vi "BatchLoad DataBuffer.vi"(0 "Display#":u16(slide)=1 min=1 max=1 step=1 scale=1.0..1.1, 7 "File Info Buffer Init":T1[](array[typedef]) {"CCD Parameters"."dt or s" format="%#.6f"; "CCD Parameters"."Repetition" min=1; "CCD Parameters"."Offset" format="%#.2f"; "CCD Parameters"."Exposure Time (s)" min=0.02 max=6000.0 format="%#.2f"; "Center nm" format="%.2f"; "Temperature (K)" format="%.2f"; "Field (T)" format="%.2f"}, 11 "Y Array In":dbl[][](array[numeric])=array1025x10[10250 elements] format="%.2f") -> (3 "File Info Out":T1={"FilePath"=path "/DATA/Labview Items", "Field (T)"=55.0, "Temperature (K)"=77.0, "X-Axis"=enum."nm", "Center nm"=55.0, "Current Grating Density"=enum."600", "CCD Parameters"={"Exposure Time (s)"=0.2, "Offset"=0.0, "BkgrdCrct"=FALSE, "Shutter"=FALSE, "Mode"=enum."Regular", "Repetition"=4, "dt or s"=0.0}, "Operation Mode"=enum."NML Data Acquisition", "Exp Index"=0, "Index_repetition"=0, "Index"=0, "Current Detector"=enum."CCD-1024x256"} {"CCD Parameters"."dt or s" format="%#.6f"; "CCD Parameters"."Repetition" min=1; "CCD Parameters"."Offset" format="%#.2f"; "CCD Parameters"."Exposure Time (s)" min=0.02 max=6000.0 format="%#.2f"; "Center nm" format="%.2f"; "Temperature (K)" format="%.2f"; "Field (T)" format="%.2f"}, 4 "X-Data out":dbl[](array[numeric]) format="%.2f", 6 "Y-Data out":dbl[](array[numeric]) format="%.2f", 8 "X-Axis":i32(ring)=1 items=["Point #", "nm", "eV", "meV", "cm-1"], 10 "File Info Buffer Out":T1[](array[typedef]) {"CCD Parameters"."dt or s" format="%#.6f"; "CCD Parameters"."Repetition" min=1; "CCD Parameters"."Offset" format="%#.2f"; "CCD Parameters"."Exposure Time (s)" min=0.02 max=6000.0 format="%#.2f"; "Center nm" format="%.2f"; "Temperature (K)" format="%.2f"; "Field (T)" format="%.2f"}, 14 "Continue?":bool, 15 "Y Array Out":dbl[][](array[numeric]) format="%.2f")   [LabVIEW 2019]
doc: "Write (FIFO) or retrieve (LIFO) data from the buffer.\n\nWhen write to the buffer, set the desired \"Buffer Size\" and run the VI several iterations. Notice that initially, the buffer grows to reach \"Buffer Size\" and then the input data flows from the last buffer element through to the zero element on each iteration (First In, First Out).\n\nWhen read from the buffer, set the Read# to the nth previous input data, i.e. counting reversely, with the most recent input counted as the 1st readout. If the input is out of current buffer size, an error is returned. (Last In, First Out)"
uses:
  Globals and TypeDefs/Type Definitions.llb/FileInfoParameter.ctt
  Globals and TypeDefs/Type Definitions.llb/Wavelength Unit.ctt
  Globals and TypeDefs/Type Definitions.llb/McPherson Grating Density.ctl
  Globals and TypeDefs/Type Definitions.llb/CCDParameter.ctt
  Globals and TypeDefs/Type Definitions.llb/OperationMode.ctt
  Globals and TypeDefs/Type Definitions.llb/ListOfDetectors.ctt
  File and save/X-Axis_Generator_morph.vi
panel:
  in  "End #":i16
  in  "Start #":i16
  in  "continue2":bool=TRUE
  in  "Speed":u16(slide)=100 min=50 max=5000 step=50 scale=10.0..5000.0
  in  "Movie":bool
  out "File Contents":string
  in  "WL unit":i32(ring)=1 items=["Wavelength", "nm", "eV", "meV", "cm-1"]
  in  "Continue?":bool
  in  "Cancel":bool
  out "File Path":path
  out "?":T7(graph)
  # "Latest"
  # "Erliest"
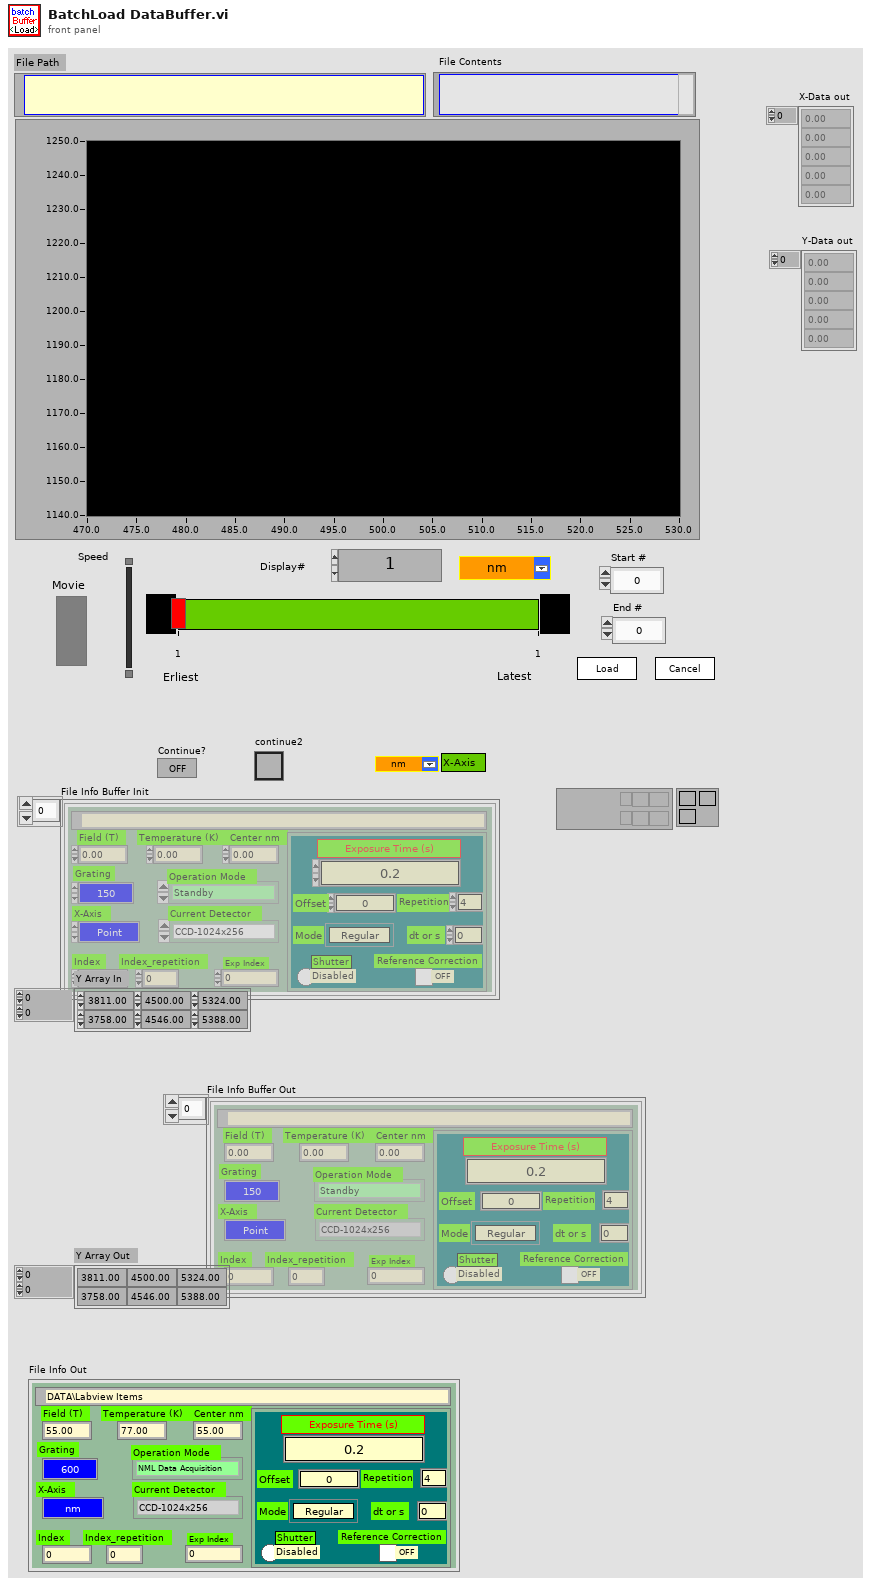
[diagram p1: front panel]
types:
  T1 = typedef "FileInfoParameter.ctt" = cluster{"FilePath":path, "Field (T)":dbl, "Temperature (K)":dbl, "X-Axis":T2, "Center nm":dbl, "Current Grating Density":T3, "CCD Parameters":T4, "Operation Mode":T5, "Exp Index":u32, "Index_repetition":u16, "Index":u16, "Current Detector":T6}
  T2 = typedef "Wavelength Unit.ctt" = enum8{"Point", "nm", "eV", "meV", "cm_1"}
  T3 = typedef "McPherson Grating Density.ctl" = enum8{"150", "300", "600", "1200", "1800"}
  T4 = typedef "CCDParameter.ctt" = cluster{"Exposure Time (s)":dbl, "Offset":dbl, "BkgrdCrct":bool, "Shutter":bool, "Mode":enum8{"Regular", "OverExp Cor", "SpikeRemove", "ForCalibration"}, "Repetition":u16, "dt or s":dbl}
  T5 = typedef "OperationMode.ctt" = enum16{"Standby", "CCD Single Shot", "CCD Sequence Shots", "CCD Custom Shots", "CCD Reference Shot", "Step Scanning ", "Time Scanning", "NML Data Acquisition"}
  T6 = typedef "ListOfDetectors.ctt" = enum8{"CCD-1024x256", "InGaAs PDA-1024x1", "CCD-1340x400", "Ge Single Channel", "Si Single Channel", "PMT Single Channel"}
  T7 = cluster{"Ramp Pattern":dbl[], "Sinc Pattern":dbl[]}
  T8 = enum16{"Pass", "Write", "Read", "ReadPlotBlock", "Initialize", "InitFromBufferInput", "Resize Buffer"}
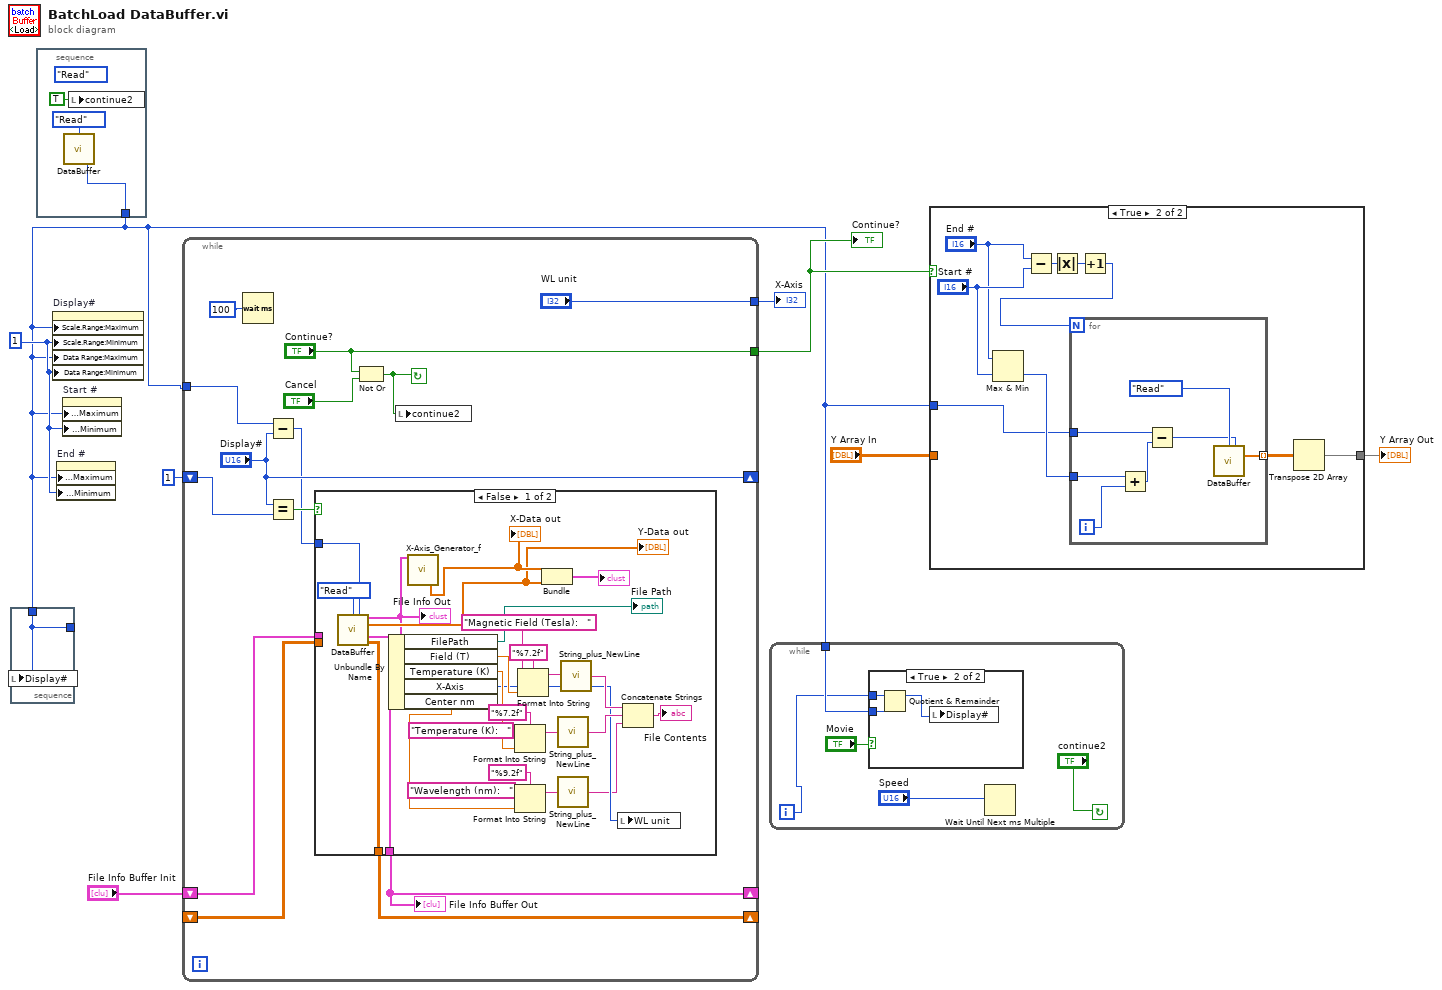
[diagram p0: block diagram]
diagram:
  w2 = u32 1 ("milliseconds to wait")
  n1 = stacked-sequence {
    tunnel: [w10] -> w1
    frame #0 {
      (unwired) enum16{"Pass", "Write", "Read", "Initialize"}."Read" ("Action")
      n2 = call "DataBuffer.vi"("Action"=T8."Read") -> ("Current Buffer Size"=w10:i32)  [unwired: 10 in, 4 out]
      n3 = local write "continue2"(TRUE ("Boolean")) -> ()
    }
  }
  n4 = stacked-sequence {
    tunnel: w1 -> [w12]
    tunnel: [w12] -> _
    frame #0 {
      n5 = local write "Display#"(w12) -> ()
    }
  }
  n6 = property on="Display#" class="Slide (strict)"("Scale.Range:Maximum"=w1, "Scale.Range:Minimum"=w2, "Data Range:Maximum"=w1, "Data Range:Minimum"=w2) -> ()  [unwired: 2 in, 2 out]
  n7 = property on="End #" class="DigNum (strict)"("Data Range:Maximum"=w1, "Data Range:Minimum"=w2) -> ()  [unwired: 2 in, 2 out]
  n8 = property on="Start #" class="DigNum (strict)"("Data Range:Maximum"=w1, "Data Range:Minimum"=w2) -> ()  [unwired: 2 in, 2 out]
  n9 = while {
    tunnel: w1 -> [w21]
    shift-left: u8 1 ("Read#") -> [w23]
    shift-right: ["Display#"] -> _
    tunnel: ["Continue?"] -> w5
    tunnel: ["WL unit"] -> w7
    shift-right: [w14] -> _
    shift-left: "File Info Buffer Init" -> [w16]
    shift-right: [w13] -> _
    shift-left: _ -> [w15]
    stop <- w18 continue-if-true
    n10 = Wait (ms)(milliseconds to wait=u32 100) -> ()  [unwired: 1 out]
    n11 = Subtract(x=w21, y="Display#") -> (x-y=w19:i32)
    n12 = Equal?(x="Display#", y=w23) -> (x = y?=w22:bool)
    n13 = case shown="False" w22 {
      tunnel: w19 -> [w42 _]
      tunnel: w16 -> [_ w54]
      tunnel: w15 -> [_ w53]
      tunnel: [w35 w54] -> w14
      tunnel: [w34 w53] -> w13
      frame False {
        n14 = call "DataBuffer.vi"("Action"=T8."Read", "Read#"=w42) -> ("File Info Out"=w39:T1, "Y Array out"=w40:dbl[], "File Info Buffer Out"=w35:T1[], "Y Array Buffer Out"=w34:dbl[][])  [unwired: 9 in, 1 out]
        "Y-Data out" <- w40
        "File Info Out" <- w39
        n15 = Unbundle By Name(w39) -> ("FilePath"=→"File Path":path, "Field (T)"=w37:dbl, "Temperature (K)"=w36:dbl, "X-Axis"=w33:T2, "Center nm"=w28:dbl)
        n16 = call-poly "X-Axis_Generator_f.vi"("File Info In"=w39) -> ("X-axis"=w41:dbl[])  [unwired: 11 in, 7 out]
        "X-Data out" <- w41
        n17 = Format Into String(format string="%7.2f", initial string="Temperature (K):   ", w36) -> (resulting string=w48:string)  [unwired: 1 in, 1 out]
        n18 = Format Into String(format string="%9.2f", initial string="Wavelength (nm):   ", w28) -> (resulting string=w31:string)  [unwired: 1 in, 1 out]
        n19 = Format Into String(format string="%7.2f", initial string="Magnetic Field (Tesla):   ", w37) -> (resulting string=w50:string)  [unwired: 1 in, 1 out]
        n20 = Bundle("X-axis"=w41, "Y Array out"=w40) -> (→"?":cluster{"X-axis":dbl[], "Y Array out":dbl[]})  [unwired: 1 in]
        n21 = call "String_plus_NewLine.vi"("Input String"=w48) -> ("Input String +[\\n]"=w44:string)
        n22 = call "String_plus_NewLine.vi"("Input String"=w31) -> ("Input String +[\\n]"=w27:string)
        n23 = call "String_plus_NewLine.vi"("Input String"=w50) -> ("Input String +[\\n]"=w45:string)
        n24 = local write "WL unit"(w33) -> ()
        n25 = Concatenate Strings(w45, w44, w27) -> (→"File Contents":string)
      }
      frame True {
      }
    }
    "File Info Buffer Out" <- w14
    n26 = Not Or(1:"Cancel", 2:"Continue?") -> (0:w18:bool)
    n27 = local write "continue2"(w18) -> ()
  }
  "Continue?" <- w5
  "X-Axis" <- w7
  n28 = while {
    tunnel: w1 -> [w59]
    i -> [w56]
    stop <- "continue2" continue-if-true
    n29 = case shown="True" "Movie" {
      tunnel: w59 -> [_ w62]
      tunnel: w56 -> [_ w60]
      frame False {
      }
      frame True {
        n30 = Quotient & Remainder(x=w60, y=w62) -> (x-y*floor(x/y)=w61:i32)  [unwired: 1 out]
        n31 = local write "Display#"(w61) -> ()
      }
    }
    n32 = Wait Until Next ms Multiple(millisecond multiple="Speed") -> ()  [unwired: 1 out]
  }
  n33 = case shown="True" w5 {
    tunnel: [w63 w64] -> w3
    tunnel: "Y Array In" -> [w63 _]
    tunnel: w1 -> [_ w66]
    frame False {
    }
    frame True {
      n34 = Max & Min(x="End #", y="Start #") -> (min(x,y)=w67:i16)  [unwired: 1 out]
      n35 = Subtract(x="End #", y="Start #") -> (x-y=w72:i16)
      n36 = Absolute Value(x=w72) -> (abs(x)=w71:i16)
      n37 = Increment(x=w71) -> (x+1=w70:i16)
      n38 = for {
        N: w70 -> [_]
        tunnel: w67 -> [w77]
        tunnel: w66 -> [w76]
        tunnel: [w73] -> w65 mode=indexing
        i -> [w78]
        n39 = Add(x=w77, y=w78) -> (x+y=w75:i32)
        n40 = Subtract(x=w76, y=w75) -> (x-y=w74:i32)
        n41 = call "DataBuffer.vi"("Action"=T8."Read", "Read#"=w74) -> ("Y Array out"=w73:dbl[])  [unwired: 9 in, 4 out]
      }
      n42 = Transpose 2D Array(2D array=w65) -> (transposed array=w64:dbl[][])
    }
  }
  "Y Array Out" <- w3
